vi "GIALAP_KIA_LABVIEW.vi"() -> ()   [LabVIEW 2020]
uses:
  <vilib>/Instr/_visa.llb/VISA Configure Serial Port (Instr).vi
panel:
  in  "Tab Control":enum32{"Page 1", "Page 2", "Page 3"}(tab)
  out "ECT":i32
  out "LOAD 2":i32
  out "TPS 2":i32
  out "IAT 2":i32
  out "MAP 2":i32
  out "ECT 2":i64(slide)=-50 scale=-50.0..150.0
  out "Toc do xe 2":i64(knob) scale=0.0..220.0
  out "Toc do dong co 2":i64(knob) scale=0.0..8000.0
  out "TOC DO XE":i32(graph)
  out "TOC DO DONG CO":i32(graph)
  in  "Clear":bool
  out "Bang len so":cluster{"Y":dbl[], "Y":dbl[]}[](graph)
  out "Bang chuyen so":cluster{"Y":dbl[], "Y":dbl[]}[](graph)
  in  "Red":u32(colorbox)=16711680
  in  "Yellow":u32(colorbox)=16775793
  in  "Green":u32(colorbox)=1244968
  out "read buffer":string="a678b95c0d0e0f0g61h16i28j\r\n"
  in  "VISA resource name":refnum<visa-resource-name>="COM7"
  in  "stop":bool
  # "kPa"
  # "°C"
  # "%"
  # "%"
  # "°C"
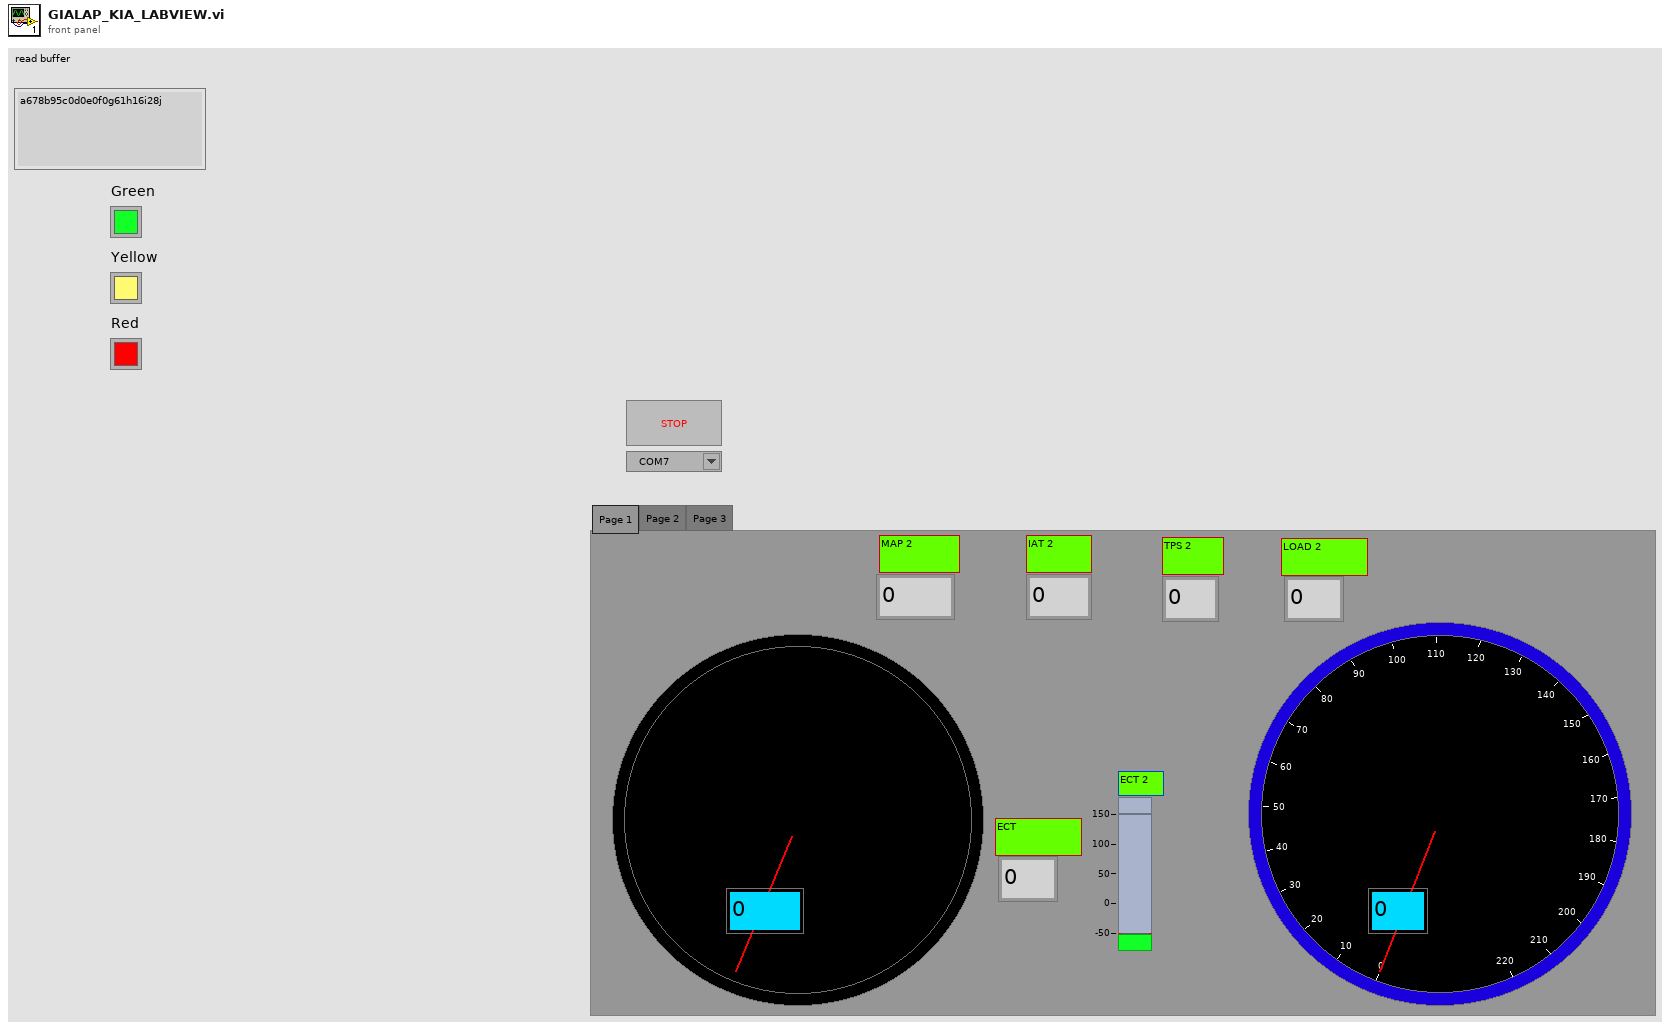
[diagram p1: front panel]
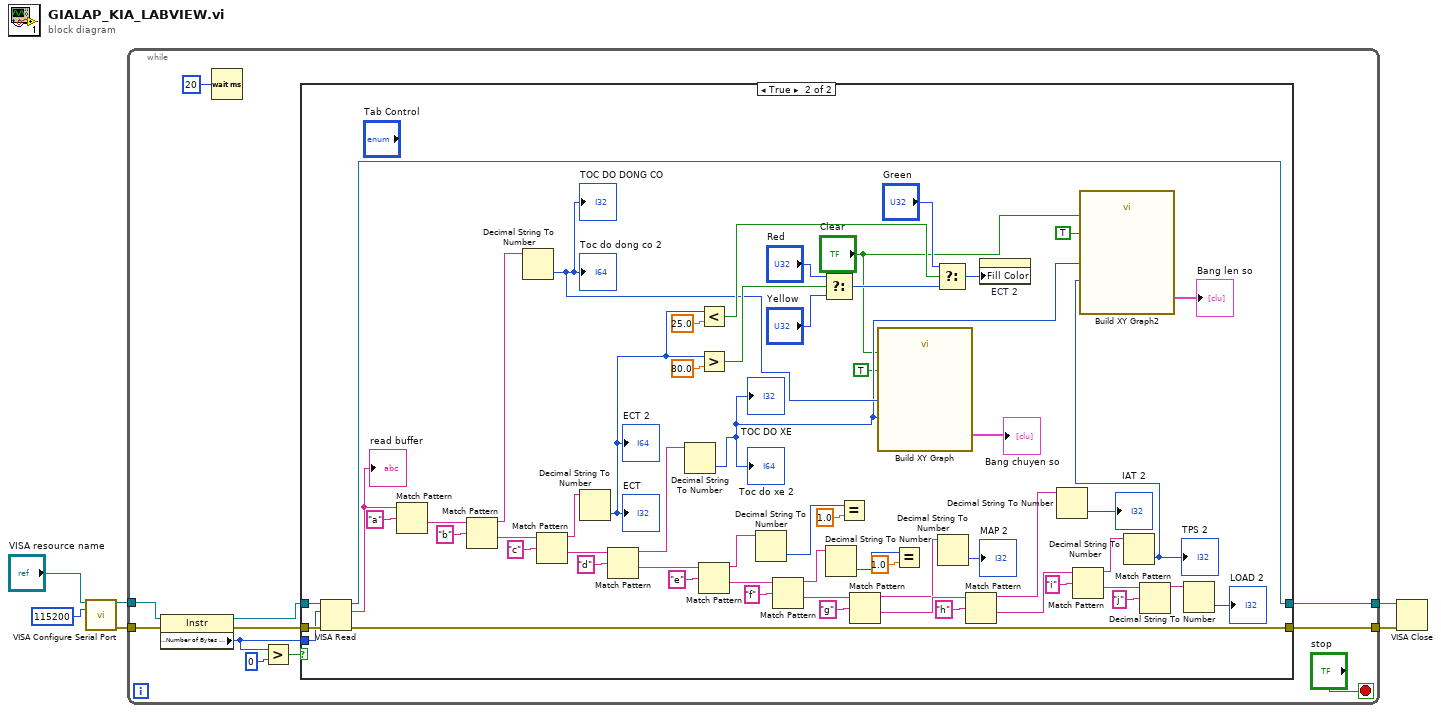
[diagram p0: block diagram]
diagram:
  n1 = call-poly "VISA Configure Serial Port"("VISA resource name"="VISA resource name", "baud rate (9600)"=u32 115200) -> ("VISA resource name out"=w4:refnum<visa-resource-name>, "error out"=w3:errorcluster)  [unwired: 12 in]
  n2 = while {
    tunnel: w4 -> [w8]
    tunnel: w3 -> [w7]
    tunnel: [w13] -> w2
    tunnel: [w12] -> w1
    stop <- "stop" stop-if-true
    n3 = property class="Instr"(reference=w8, error in=w7) -> (reference out=w15:refnum<visa-resource-name>, error out=w14:errorcluster, "Serial Settings:Number of Bytes at Serial Port"=w10:u32)
    n4 = Wait (ms)(milliseconds to wait=u32 20) -> ()  [unwired: 1 out]
    n5 = Greater?(x=w10, y=u32 0) -> (0:w11:bool)
    n6 = case shown="True" w11 {
      tunnel: w15 -> [w19 w78]
      tunnel: w14 -> [w18 w77]
      tunnel: [w19 w76] -> w13
      tunnel: [w18 w75] -> w12
      tunnel: w10 -> [_ w74]
      frame False {
      }
      frame True {
        n7 = VISA Read(VISA resource name=w78, byte count=w74, error in (no error)=w77) -> (VISA resource name out=w76:refnum<visa-resource-name>, read buffer=w73:string, error out=w75:errorcluster)  [unwired: 1 out]
        "read buffer" <- w73
        n8 = Match Pattern(string=w73, regular expression="a") -> (after substring=w70:string)  [unwired: 1 in, 3 out]
        n9 = Match Pattern(string=w70, regular expression="b") -> (before substring=w67:string, after substring=w68:string)  [unwired: 1 in, 2 out]
        n10 = Decimal String To Number(string=w67) -> (number=w26:i32)  [unwired: 2 in, 1 out]
        "Toc do dong co 2" <- w26
        "TOC DO DONG CO" <- w26
        n11 = Match Pattern(string=w68, regular expression="c") -> (before substring=w66:string, after substring=w65:string)  [unwired: 1 in, 2 out]
        n12 = Decimal String To Number(string=w66) -> (number=w28:i32)  [unwired: 2 in, 1 out]
        "ECT 2" <- w28
        "ECT" <- w28
        n13 = Match Pattern(string=w65, regular expression="d") -> (before substring=w63:string, after substring=w43:string)  [unwired: 1 in, 2 out]
        n14 = Decimal String To Number(string=w63) -> (number=w24:i32)  [unwired: 2 in, 1 out]
        "Toc do xe 2" <- w24
        "TOC DO XE" <- w24
        n15 = Less?(x=w28, y=25.0) -> (x < y?=w59:bool)
        n16 = Greater?(x=w28, y=80.0) -> (0:w57:bool)
        n17 = Match Pattern(string=w43, regular expression="e") -> (before substring=w42:string, after substring=w48:string)  [unwired: 1 in, 2 out]
        n18 = Decimal String To Number(string=w42) -> (number=w35:i32)  [unwired: 2 in, 1 out]
        n19 = Match Pattern(string=w48, regular expression="f") -> (before substring=w41:string, after substring=w47:string)  [unwired: 1 in, 2 out]
        n20 = Select(t="Red", s=w57, f="Yellow") -> (s? t:f=w55:u32)
        n21 = Decimal String To Number(string=w41) -> (number=w33:i32)  [unwired: 2 in, 1 out]
        n22 = Equal?(x=w35, y=1.0) -> ()  [unwired: 1 out]
        n23 = Match Pattern(string=w47, regular expression="g") -> (before substring=w40:string, after substring=w46:string)  [unwired: 1 in, 2 out]
        n24 = call "Build XY Graph"("Enable"=TRUE, "Reset"="Clear", "Y Input"=w24, "X Input"=w26) -> ("XY Graph"=→"Bang chuyen so":cluster{"X":dbl[], "Y":dbl[]}[])  [unwired: 6 in, 1 out]
        n25 = Equal?(x=w33, y=1.0) -> ()  [unwired: 1 out]
        n26 = Select(t="Green", s=w59, f=w55) -> (s? t:f=w29:u32)
        n27 = Decimal String To Number(string=w40) -> (number=→"MAP 2":i32)  [unwired: 2 in, 1 out]
        n28 = Match Pattern(string=w46, regular expression="h") -> (before substring=w39:string, after substring=w45:string)  [unwired: 1 in, 2 out]
        n29 = property on="ECT 2" class="Slide (strict)"("Fill Color"=w29) -> ()  [unwired: 2 in, 2 out]
        n30 = Decimal String To Number(string=w39) -> (number=→"IAT 2":i32)  [unwired: 2 in, 1 out]
        n31 = Match Pattern(string=w45, regular expression="i") -> (before substring=w38:string, after substring=w44:string)  [unwired: 1 in, 2 out]
        n32 = Decimal String To Number(string=w38) -> (number=w23:i32)  [unwired: 2 in, 1 out]
        "TPS 2" <- w23
        n33 = call "Build XY Graph2"("Enable"=TRUE, "Reset"="Clear", "Y Input"=w23, "X Input"=w24) -> ("XY Graph"=→"Bang len so":cluster{"X":dbl[], "Y":dbl[]}[])  [unwired: 6 in, 1 out]
        n34 = Match Pattern(string=w44, regular expression="j") -> (before substring=w37:string)  [unwired: 1 in, 3 out]
        n35 = Decimal String To Number(string=w37) -> (number=→"LOAD 2":i32)  [unwired: 2 in, 1 out]
      }
    }
  }
  n36 = VISA Close(VISA resource name=w2, error in (no error)=w1) -> ()  [unwired: 1 out]
